vi "S2C_ExeScriptTestRoute.vi"(7 "Q_Ref":refnum<queue>, 8 "Error In":errorcluster) -> (0 "Error Out":errorcluster)   [LabVIEW 2015]
doc: "Update the results cell in the execution table for the currently executing line item, and determines the next step to take in the execution."
uses:
  Globals/S2C_Globals.vi
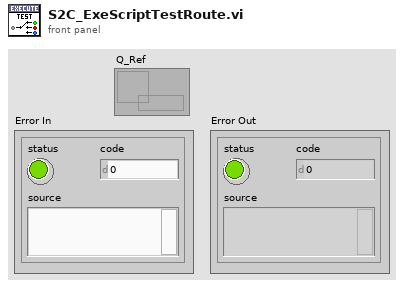
[diagram p1: front panel]
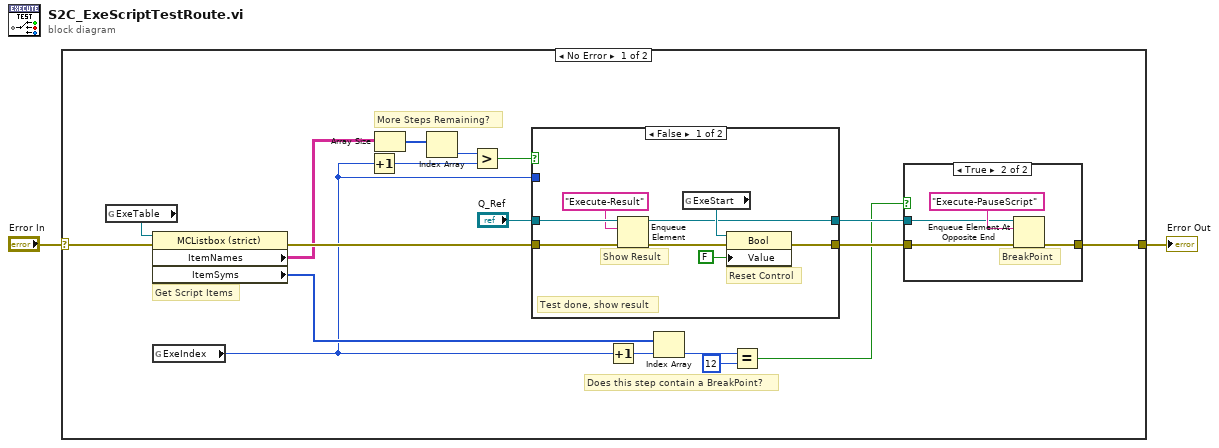
[diagram p0: block diagram]
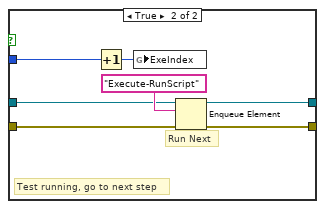
[diagram p3: hidden frame]
diagram:
  n1 = case shown="No Error" "Error In" {
    selector: "Error In" -> [w13 w41]
    tunnel: [w15 w41] -> w1
    frame No Error {
      # "Does this step contain a BreakPoint?"
      # "Get Script Items"
      # "More Steps Remaining?"
      n2 = global read "S2C_Globals.vi" "ExeTable"() -> (w14:refnum<vi>)
      n3 = property class="MCListbox (strict)"(reference=w14, error in=w13) -> (error out=w8:errorcluster, "ItemNames"=w5:string[][], "ItemSyms"=w9:i32[])  [unwired: 1 out]
      n4 = global read "S2C_Globals.vi" "ExeIndex"() -> (w3:i32)
      n5 = Increment(x=w3) -> (x+1=w17:i32)
      n6 = Array Size(array=w5) -> (size(s)=w19:i32[])
      n7 = Index Array(array=w19) -> (element=w18:i32)  [unwired: 1 in]
      n8 = Greater?(x=w18, y=w17) -> (0:w16:bool)
      n9 = case shown="False" w16 {
        tunnel: w3 -> [_ w36]
        tunnel: w8 -> [w30 w40]
        tunnel: [w32 w39] -> w7
        tunnel: "Q_Ref" -> [w29 w35]
        tunnel: [w26 w34] -> w6
        frame False {
          # "Test done, show result"
          # "Show Result"
          # "Reset Control"
          n10 = Enqueue Element(queue=w29, element="Execute-Result", error in (no error)=w30) -> (queue out=w26:refnum<queue>, error out=w28:errorcluster)  [unwired: 1 in, 1 out]
          n11 = global read "S2C_Globals.vi" "ExeStart"() -> (w33:refnum<vi>)
          n12 = property class="Bool"(reference=w33, error in=w28, "Value"=FALSE) -> (error out=w32:errorcluster)  [unwired: 1 out]
        }
        frame True {
          # "Test running, go to next step"
          # "Run Next"
          n13 = Increment(x=w36) -> (x+1=w37:i32)
          n14 = global write "S2C_Globals.vi" "ExeIndex"(w37) -> ()
          n15 = Enqueue Element(queue=w35, element="Execute-RunScript", error in (no error)=w40) -> (queue out=w34:refnum<queue>, error out=w39:errorcluster)  [unwired: 1 in, 1 out]
        }
      }
      n16 = Increment(x=w3) -> (x+1=w12:i32)
      n17 = Index Array(array=w9, index=w12) -> (element=w10:i32)
      n18 = Equal?(x=w10, y=12) -> (x = y?=w4:bool)
      n19 = case shown="True" w4 {
        tunnel: w7 -> [w21 w24]
        tunnel: [w21 w23] -> w15
        tunnel: w6 -> [_ w22]
        frame False {
        }
        frame True {
          # "BreakPoint"
          n20 = Enqueue Element At Opposite End(queue=w22, element="Execute-PauseScript", error in (no error)=w24) -> (error out=w23:errorcluster)  [unwired: 1 in, 2 out]
        }
      }
    }
    frame Error {
    }
  }
  "Error Out" <- w1
